vi "Arrange VIWin - Arrange Other FP Objects.vi"(0 "VI in":refnum<vi>, 1 "FP objects arrangement info":T1, 5 "controls from conn pane":refnum<vi>[](array[refnum]), 7 "max bottom of arranged controls":i16, 11 "error in":errorcluster) -> (15 "error out":errorcluster)   [LabVIEW 2012, in "Arrange VI Window.lvlib"]
uses:
  Arrange VI Window.lvlib
  Arrange VIWin - FP Objects Arrangement Info.ctl
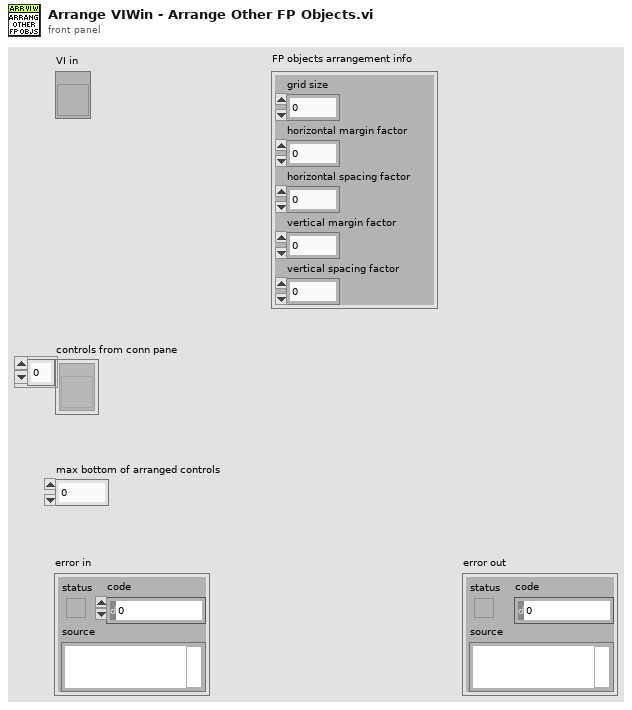
[diagram p1: front panel]
types:
  T1 = typedef "Arrange VI Window.lvlib/Arrange VIWin - FP Objects Arrangement Info.ctl" = cluster{"grid size":i32, "horizontal margin factor":i32, "horizontal spacing factor":i32, "vertical margin factor":i32, "vertical spacing factor":i32}
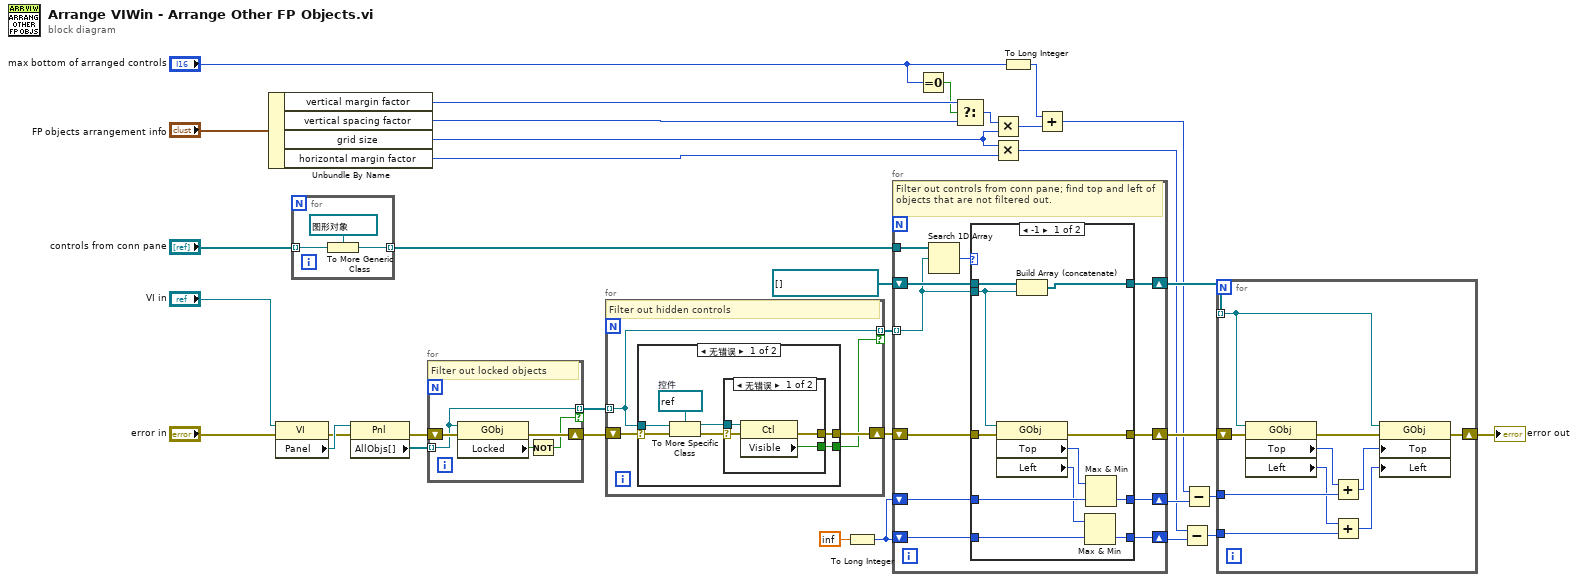
[diagram p0: block diagram]
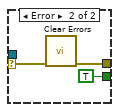
[diagram p2: hidden frame]
diagram:
  n1 = Unbundle By Name("FP objects arrangement info") -> ("vertical margin factor"=w15:i32, "vertical spacing factor"=w14:i32, "grid size"=w20:i32, "horizontal margin factor"=w21:i32)
  n2 = property class="VI"(reference="VI in", error in="error in") -> (error out=w30:errorcluster, "Panel"=w31:refnum<vi>)  [unwired: 1 out]
  n3 = for {
    tunnel: "controls from conn pane" -> [w37] mode=indexing
    tunnel: [w36] -> w4 mode=indexing
    n4 = To More Generic Class(target class=refnum<vi> refnum, reference=w37) -> (generic class reference=w36:refnum<vi>)
  }
  n5 = property class="Pnl"(reference=w31, error in=w30) -> (error out=w10:errorcluster, "AllObjs[]"=w9:refnum<vi>[])  [unwired: 1 out]
  n6 = for {
    shift-right: [w41] -> w3
    shift-left: w10 -> [w42]
    tunnel: w9 -> [w40] mode=indexing
    tunnel: [w40] -> w8 mode=indexing if=w39
    # "Filter out locked objects"
    n7 = property class="GObj"(reference=w40, error in=w42) -> (error out=w41:errorcluster, "Locked"=w38:bool)  [unwired: 1 out]
    n8 = Not(x=w38) -> (.not. x?=w39:bool)
  }
  n9 = for {
    tunnel: w8 -> [w45] mode=indexing
    shift-right: [w46] -> w7
    shift-left: w3 -> [w43]
    tunnel: [w45] -> w6 mode=indexing if=w44
    # "Filter out hidden controls"
    n10 = case shown="无错误" w43 {
      selector: w43 -> [w53 w61]
      tunnel: w45 -> [w52 _]
      tunnel: [w49 w61] -> w46
      tunnel: [w47 _] -> w44
      frame No Error {
        w51 = refnum<vi> refnum  # 控件
        n11 = To More Specific Class(target class=w51, reference=w52, error in=w53) -> (specific class reference=w48:refnum<vi>, error out=w50:errorcluster)
        n12 = case shown="无错误" w50 {
          selector: w50 -> [w57 w60]
          tunnel: [w56 w58] -> w49
          tunnel: w48 -> [w55 _]
          tunnel: [w54 TRUE ("Visible")] -> w47
          frame No Error {
            n13 = property class="Ctl"(reference=w55, error in=w57) -> (error out=w56:errorcluster, "Visible"=w54:bool)  [unwired: 1 out]
          }
          frame Error {
            n14 = call <vilib>:"Clear Errors.vi"("error in (no error)"=w60) -> ("error out"=w58:errorcluster)  [unwired: 6 in]
          }
        }
      }
      frame Error {
      }
    }
  }
  n15 = To Long Integer(number=inf) -> (32bit integer=w22:i32)
  n16 = for {
    shift-right: [w69] -> w28
    shift-left: w7 -> [w72]
    tunnel: w4 -> [w71]
    shift-right: [w67] -> w24
    shift-left: refnum<vi>[] [] ("All Objects[]") -> [w68]
    shift-right: [w65] -> w25
    shift-left: w22 -> [w66]
    shift-right: [w64] -> w18
    shift-left: w22 -> [w63]
    tunnel: w6 -> [w62] mode=indexing
    # "Filter out controls from conn pane; find top and left of objects that are not filtered out."
    n17 = Search 1D Array(1D array=w71, element=w62) -> (index of element=w70:i32)  [unwired: 1 in]
    n18 = case shown="-1" w70 {
      tunnel: w72 -> [w83 w87]
      tunnel: w62 -> [w81 _]
      tunnel: [w76 w87] -> w69
      tunnel: w68 -> [w82 w86]
      tunnel: [w80 w86] -> w67
      tunnel: w66 -> [w79 w85]
      tunnel: [w78 w85] -> w65
      tunnel: [w75 w84] -> w64
      tunnel: w63 -> [w73 w84]
      frame -1 {
        n19 = property class="GObj"(reference=w81, error in=w83) -> (error out=w76:errorcluster, "Top"=w77:i32, "Left"=w74:i32)  [unwired: 1 out]
        n20 = Build Array (concatenate)(w82, w81) -> (w80:refnum<vi>[])
        n21 = Max & Min(x=w74, y=w73) -> (min(x,y)=w75:i32)  [unwired: 1 out]
        n22 = Max & Min(x=w77, y=w79) -> (min(x,y)=w78:i32)  [unwired: 1 out]
      }
      frame Default {
      }
    }
  }
  n23 = Equal To 0?(x="max bottom of arranged controls") -> (x = 0?=w12:bool)
  n24 = Select(t=w15, s=w12, f=w14) -> (s? t:f=w13:i32)
  n25 = Multiply(x=w13, y=w20) -> (x*y=w27:i32)
  n26 = Multiply(x=w20, y=w21) -> (x*y=w19:i32)
  n27 = To Long Integer(number="max bottom of arranged controls") -> (32bit integer=w26:i32)
  n28 = Add(x=w26, y=w27) -> (x+y=w16:i32)
  n29 = Subtract(x=w19, y=w18) -> (x-y=w17:i32)
  n30 = Subtract(x=w16, y=w25) -> (x-y=w5:i32)
  n31 = for {
    shift-right: [w96] -> w34
    shift-left: w28 -> [w97]
    tunnel: w24 -> [w93] mode=indexing
    tunnel: w5 -> [w94]
    tunnel: w17 -> [w91]
    n32 = property class="GObj"(reference=w93, error in=w97) -> (error out=w95:errorcluster, "Top"=w89:i32, "Left"=w92:i32)  [unwired: 1 out]
    n33 = Add(x=w89, y=w94) -> (x+y=w88:i32)
    n34 = Add(x=w92, y=w91) -> (x+y=w90:i32)
    n35 = property class="GObj"(reference=w93, error in=w95, "Top"=w88, "Left"=w90) -> (error out=w96:errorcluster)  [unwired: 1 out]
  }
  "error out" <- w34
